vi "getStatus.vi"(8 "error in (no error)":errorcluster, 11 "RSeries_CAM in":refnum<class "RSeries_CAM.lvclass">) -> (0 "error out":errorcluster, 1 "Status":string, 2 "Success?":bool, 3 "RSeries_CAM out":refnum<class "RSeries_CAM.lvclass">)   [LabVIEW 2024, in "RSeries_CAM.lvlib" / "RSeries_CAM.lvclass"]
uses:
  RSeries_CAM.lvclass
  <vilib>/Utility/error.llb/Trim Whitespace One-Sided.vi
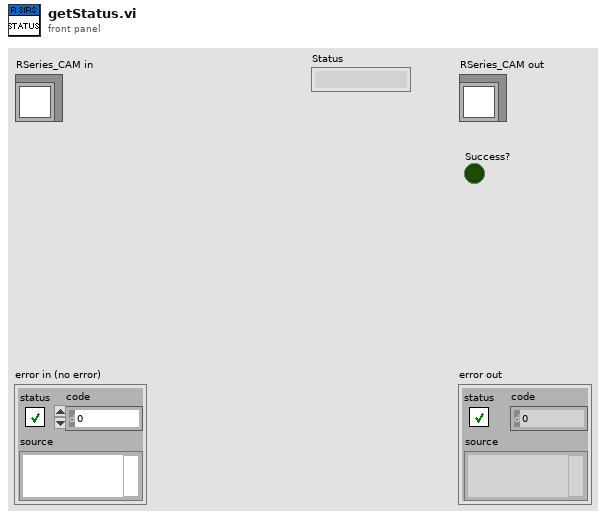
[diagram p1: front panel]
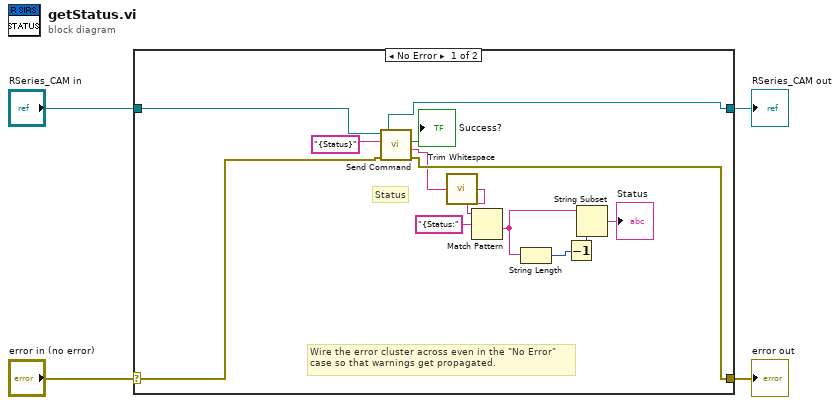
[diagram p0: block diagram]
diagram:
  n1 = case shown="No Error" "error in (no error)" {
    selector: "error in (no error)" -> [w13 w19]
    tunnel: [w12 w19] -> w3
    tunnel: [w16 w18] -> w1
    tunnel: "RSeries_CAM in" -> [w17 w18]
    frame No Error {
      # "Status"
      # "Wire the error cluster across even in the \"No Error\"\ncase so that warnings get propagated."
      n2 = call "Send Command.vi"("error in (no error)"=w13, "Command"="{Status}", "RSeries_CAM in"=w17) -> ("error out"=w12:errorcluster, "Response"=w7:string, "Success?"=→"Success?":bool, "RSeries_CAM out"=w16:refnum<class "RSeries_CAM.lvclass">)  [unwired: 5 in]
      n3 = call <vilib>:"Trim Whitespace.vi"("string"=w7) -> ("trimmed string"=w6:string)  [unwired: 1 in]
      n4 = Match Pattern(string=w6, regular expression="{Status:") -> (after substring=w8:string)  [unwired: 1 in, 3 out]
      n5 = String Length(string=w8) -> (length=w10:i32)
      n6 = Decrement(x=w10) -> (x-1=w9:i32)
      n7 = String Subset(string=w8, length (rest)=w9) -> (substring=→"Status":string)  [unwired: 1 in]
    }
    frame Error {
    }
  }
  "error out" <- w3
  "RSeries_CAM out" <- w1
